vi "myRIO_BRig_RT__Case_Exp_subState_LC__initTrial_subunit1_reward.vi"(0 "input_LR_OnOff":bool, 1 "input_I_rewarded":bool, 2 "input_I_firstTrial":bool, 3 "input_spout":u16, 4 "input_randomNumber":u16, 5 "input_LR_Block":u16, 7 "input_LR_Trial":u16, 9 "input_LR_Probability":u16) -> (8 "output_LR_Event":bool, 10 "output_LR_Laser":bool)   [LabVIEW 2014]
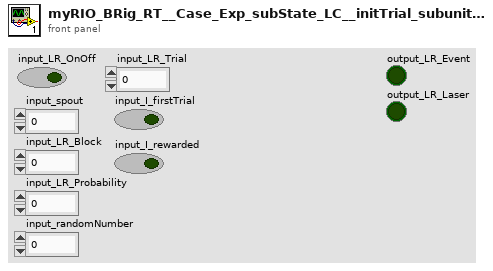
[diagram p1: front panel]
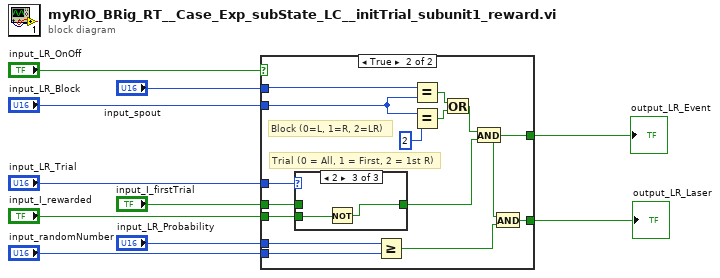
[diagram p0: block diagram]
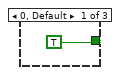
[diagram p3: hidden frame]
diagram:
  n1 = case shown="True" "input_LR_OnOff" {
    tunnel: "input_LR_Block" -> [_ w21]
    tunnel: "input_LR_Trial" -> [_ w15]
    tunnel: "input_LR_Probability" -> [_ w22]
    tunnel: [_ w18] -> w1
    tunnel: [_ w17] -> w2
    tunnel: "input_spout" -> [_ w16]
    tunnel: "input_I_rewarded" -> [_ w12]
    tunnel: "input_I_firstTrial" -> [_ w14]
    tunnel: "input_randomNumber" -> [_ w11]
    frame False {
    }
    frame True {
      # "Block (0=L, 1=R, 2=LR)"
      # "Trial (0 = All, 1 = First, 2 = 1st R)"
      n2 = case shown="2" w15 {
        tunnel: w14 -> [_ w27 _]
        tunnel: [TRUE w27 w28] -> w13
        tunnel: w12 -> [_ _ w29]
        frame 0, Default {
        }
        frame 1 {
        }
        frame 2 {
          n3 = Not(x=w29) -> (.not. x?=w28:bool)
        }
      }
      n4 = Greater Or Equal?(x=w22, y=w11) -> (x >= y?=w20:bool)
      n5 = Equal?(x=w16, y=w21) -> (x = y?=w24:bool)
      n6 = Equal?(x=w21, y=u16 2) -> (x = y?=w23:bool)
      n7 = Or(x=w24, y=w23) -> (x .or. y?=w19:bool)
      n8 = And(x=w19, y=w13) -> (x .and. y?=w17:bool)
      n9 = And(x=w17, y=w20) -> (x .and. y?=w18:bool)
    }
  }
  "output_LR_Event" <- w2
  "output_LR_Laser" <- w1
